vi "String.vi"() -> ()   [LabVIEW 2020]
panel:
  out "concatenated string 2":string
  in  "Slide":u8(slide) scale=0.0..100.0
  in  "Boolean 2":bool
  in  "Thermometer":dbl(slide) scale=0.0..100.0
  out "s? t:f":string
  in  "Boolean":bool
  in  "INDIQUE Nombre":string
  in  "INDIQUE APELLIDO":string
  out "all lower case string":string
  out "all upper case string":string
  out "substring":string
  in  "length (rest)":i32
  in  "offset (0)":i32
  out "concatenated string":string
  out "length":i32
  out "RX":string
  in  "TX":string
  # "STRING"
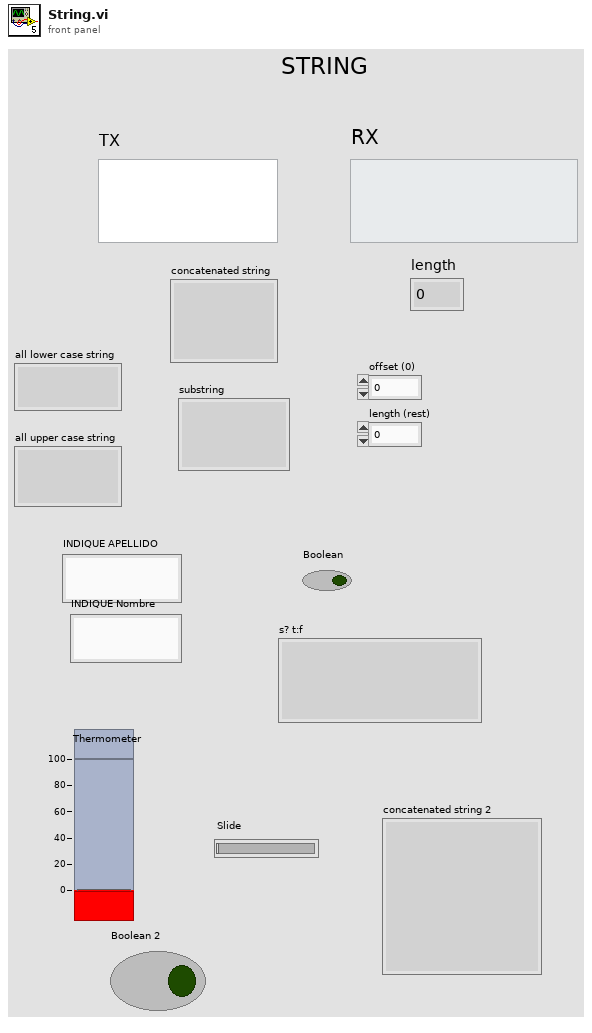
[diagram p1: front panel]
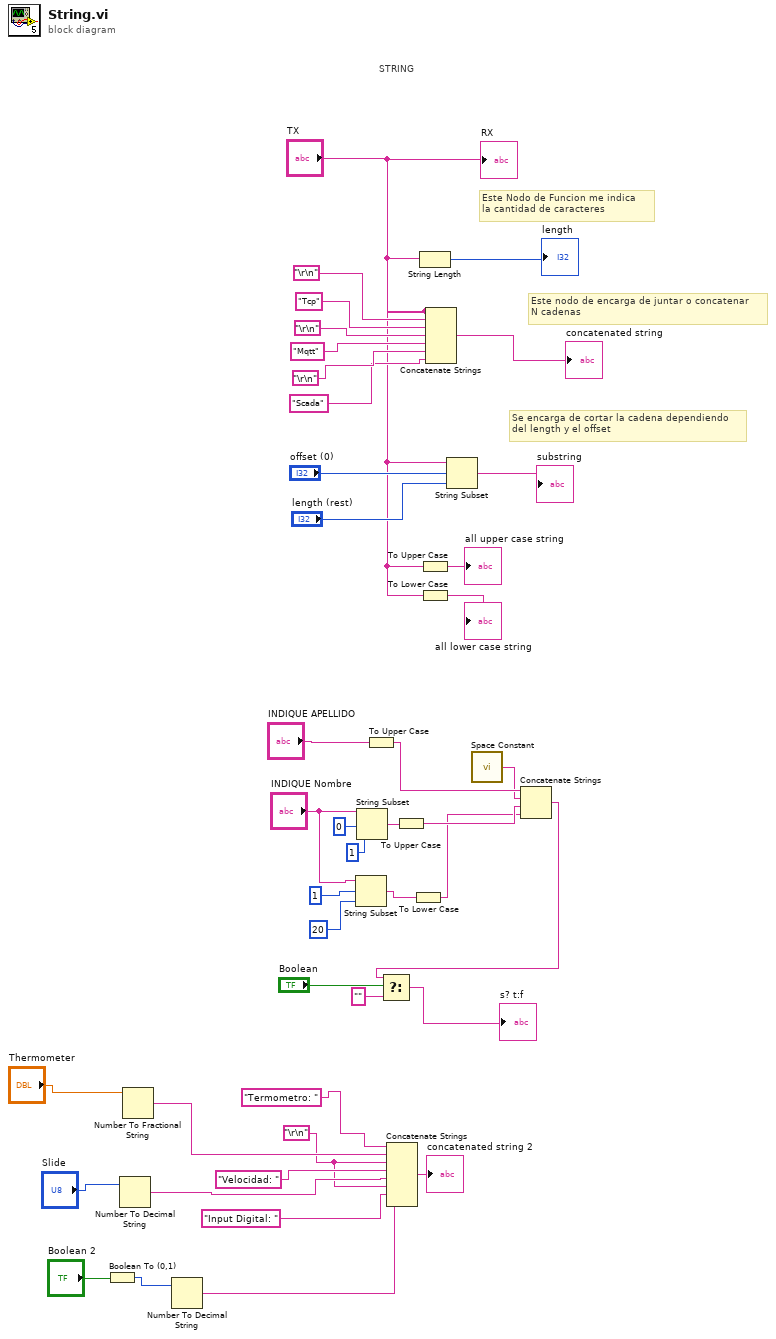
[diagram p0: block diagram]
diagram:
  w4 = "\r\n"
  # "Se encarga de cortar la cadena dependiendo\ndel length y el offset"
  # "Este nodo de encarga de juntar o concatenar\nN cadenas"
  # "Este Nodo de Funcion me indica\nla cantidad de caracteres"
  # "STRING"
  n1 = Boolean To (0,1)(Boolean="Boolean 2") -> (0, 1=w11:i16)
  n2 = Number To Decimal String(number="Slide") -> (decimal integer string=w5:string)  [unwired: 1 in]
  n3 = Number To Fractional String(number="Thermometer") -> (F-format string=w7:string)  [unwired: 3 in]
  n4 = Number To Decimal String(number=w11) -> (decimal integer string=w2:string)  [unwired: 1 in]
  n5 = String Subset(string="INDIQUE Nombre", offset (0)=1, length (rest)=20 ("length (rest)")) -> (substring=w15:string)
  n6 = String Subset(string="INDIQUE Nombre", offset (0)=0, length (rest)=1 ("length (rest)")) -> (substring=w24:string)
  n7 = To Upper Case(1:"INDIQUE APELLIDO") -> (0:w21:string)
  n8 = Concatenate Strings("Termometro: ", w7, w4, "Velocidad: ", w5, w4, "Input Digital: ", w2) -> (→"concatenated string 2":string)
  n9 = To Upper Case(1:w24) -> (0:w20:string)
  n10 = To Lower Case(string=w15) -> (all lower case string=w14:string)
  n11 = String Length(string="TX") -> (length=→"length":i32)
  n12 = To Upper Case(1:"TX") -> (0:→"all upper case string":string)
  n13 = To Lower Case(string="TX") -> (all lower case string=→"all lower case string":string)
  n14 = Concatenate Strings("TX", "\r\n", "Tcp", "\r\n", "Mqtt", "\r\n", "Scada") -> (→"concatenated string":string)
  n15 = String Subset(string="TX", offset (0)="offset (0)", length (rest)="length (rest)") -> (substring=→"substring":string)
  n16 = call <vilib>:"Space Constant.vi"() -> ("String"=w13:string)
  n17 = Concatenate Strings(w21, w13, w20, w14) -> (w18:string)
  n18 = Select(t=w18, s="Boolean", f="") -> (s? t:f=→"s? t:f":string)
  "RX" <- "TX"
